vi "Flock_Logger_Print To Console.vi"(8 "Error In":errorcluster, 10 "Text":string) -> (0 "Error Out":errorcluster, 2 "TextOut":string)   [LabVIEW 2014, in "Logger.lvlib"]
doc: "This VI checks if the VI is running on RT. If so it will print the DebugStatus message to the console."
uses:
  Logger.lvlib
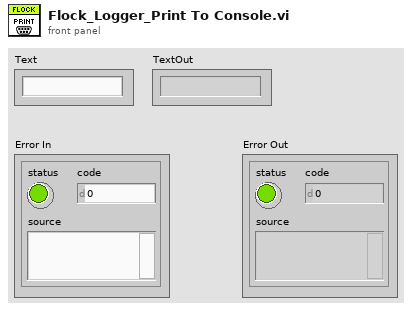
[diagram p1: front panel]
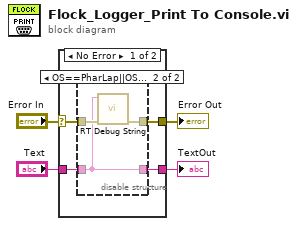
[diagram p0: block diagram]
diagram:
  n1 = case shown="No Error" "Error In" {
    selector: "Error In" -> [w8 w14]
    tunnel: [w7 w14] -> w3
    tunnel: "Text" -> [w6 _]
    tunnel: [w5 _] -> w1
    frame No Error {
      n2 = disable-structure shown="OS==PharLap||OS==VxWorks" {
        disable-tunnel: w6 -> [w10 w11]
        disable-tunnel: w8 -> [w9 w13]
        disable-tunnel: [w9 w12] -> w7
        disable-tunnel: [w10 w11] -> w5
        frame condition #0 (active) {
        }
        frame condition #1 {
          n3 = call <vilib>:"RT Debug String.vi"("error in (no error)"=w13, "String to write"=w11) -> ("error out"=w12:errorcluster)  [unwired: 9 in]
        }
      }
    }
    frame Error {
    }
  }
  "Error Out" <- w3
  "TextOut" <- w1
